vi "Open ASCII Text File.vi"() -> ()   [LabVIEW 2011]
uses:
  <vilib>/Utility/file.llb/Read From Spreadsheet File (DBL).vi
panel:
  out "deleted portion":dbl[][](array[numeric])
  in  "delimiter (\\t)":string="\t"
  out "all rows":dbl[][](array[numeric]) format="%0.3f"
  in  "file path (dialog if empty)":path
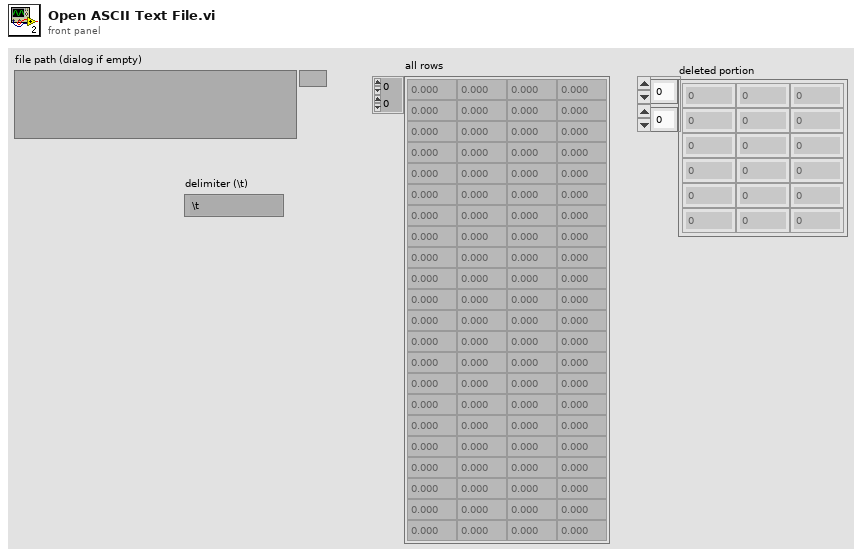
[diagram p1: front panel]
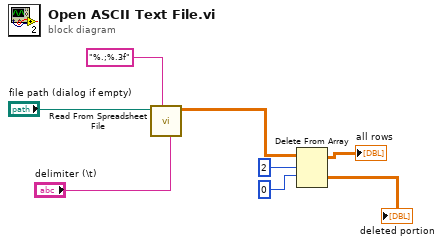
[diagram p0: block diagram]
diagram:
  n1 = call-poly <vilib>:"Read From Spreadsheet File.vi"("delimiter (\\t)"="delimiter (\\t)", "format (%.3f)"="%.;%.3f", "file path (dialog if empty)"="file path (dialog if empty)") -> ("all rows"=w5:dbl[][])  [unwired: 4 in, 4 out]
  n2 = Delete From Array(array=w5, length=2, index (row)=0) -> (deleted portion=→"deleted portion":dbl[][], array with subset deleted=→"all rows":dbl[][])  [unwired: 1 in]
